vi "detect circles 4.vi"() -> ()   [LabVIEW 2020]
uses:
  <vilib>/vision/NI_Vision_Development_Module.lvlib
panel:
  out "Distances":sgl[](array[numeric]) format="%.4f"
  out "min value":dbl
  out "Array 2":dbl[](array[numeric])
  out "Array":cdb[](array[numeric])
  out "Coordinates":i32[](array[numeric])
  out "Last Mouse Position:All Elements":cluster{"X":i32, "Y":i32}
  out "Circles Data (calibrated)":T1(array[cluster])
  in  "Operation":T2(ring)
  out "Circles Data 2":T1(array[cluster])
  out "error out":errorcluster
  out "Image IN 3":T3(plugin-control)
  in  "WindowSize":i32=9
  in  "LThres":sgl=0.2
  in  "HThresh":sgl=0.7
  in  "Sigma":sgl=1.0
  out "Circles Data":T1(array[cluster])
  in  "Detect circles":bool
  out "Y Resolution":i32
  out "X Resolution":i32
  out "Unit":T4
  out "Image Type":T5 items=["Grayscale (U8)", "Grayscale (I16)", "Grayscale (SGL)", "Complex (CSG)", "RGB (U32)", "HSL (U32)", "RGB (U64)", "Grayscale (U16)"]
  out "Image IN 2":T3(plugin-control)
  out "Image IN":T3(plugin-control)
  in  "Vertical Pointer Slide":cluster{"Numeric":dbl, "Numeric":dbl}(slide)={"Numeric"=0.0, "Numeric"=2.7353463587921847} scale=0.0..255.0
  in  "stop":bool
  in  "Image Type (Conversion 1)":T5 items=["Grayscale (U8)", "Grayscale (I16)", "Grayscale (SGL)", "Complex (CSG)", "RGB (U32)", "HSL (U32)", "RGB (U64)", "Grayscale (U16)"]
  in  "Bit Depth (Original Image)":u32=15
  in  "error in":errorcluster
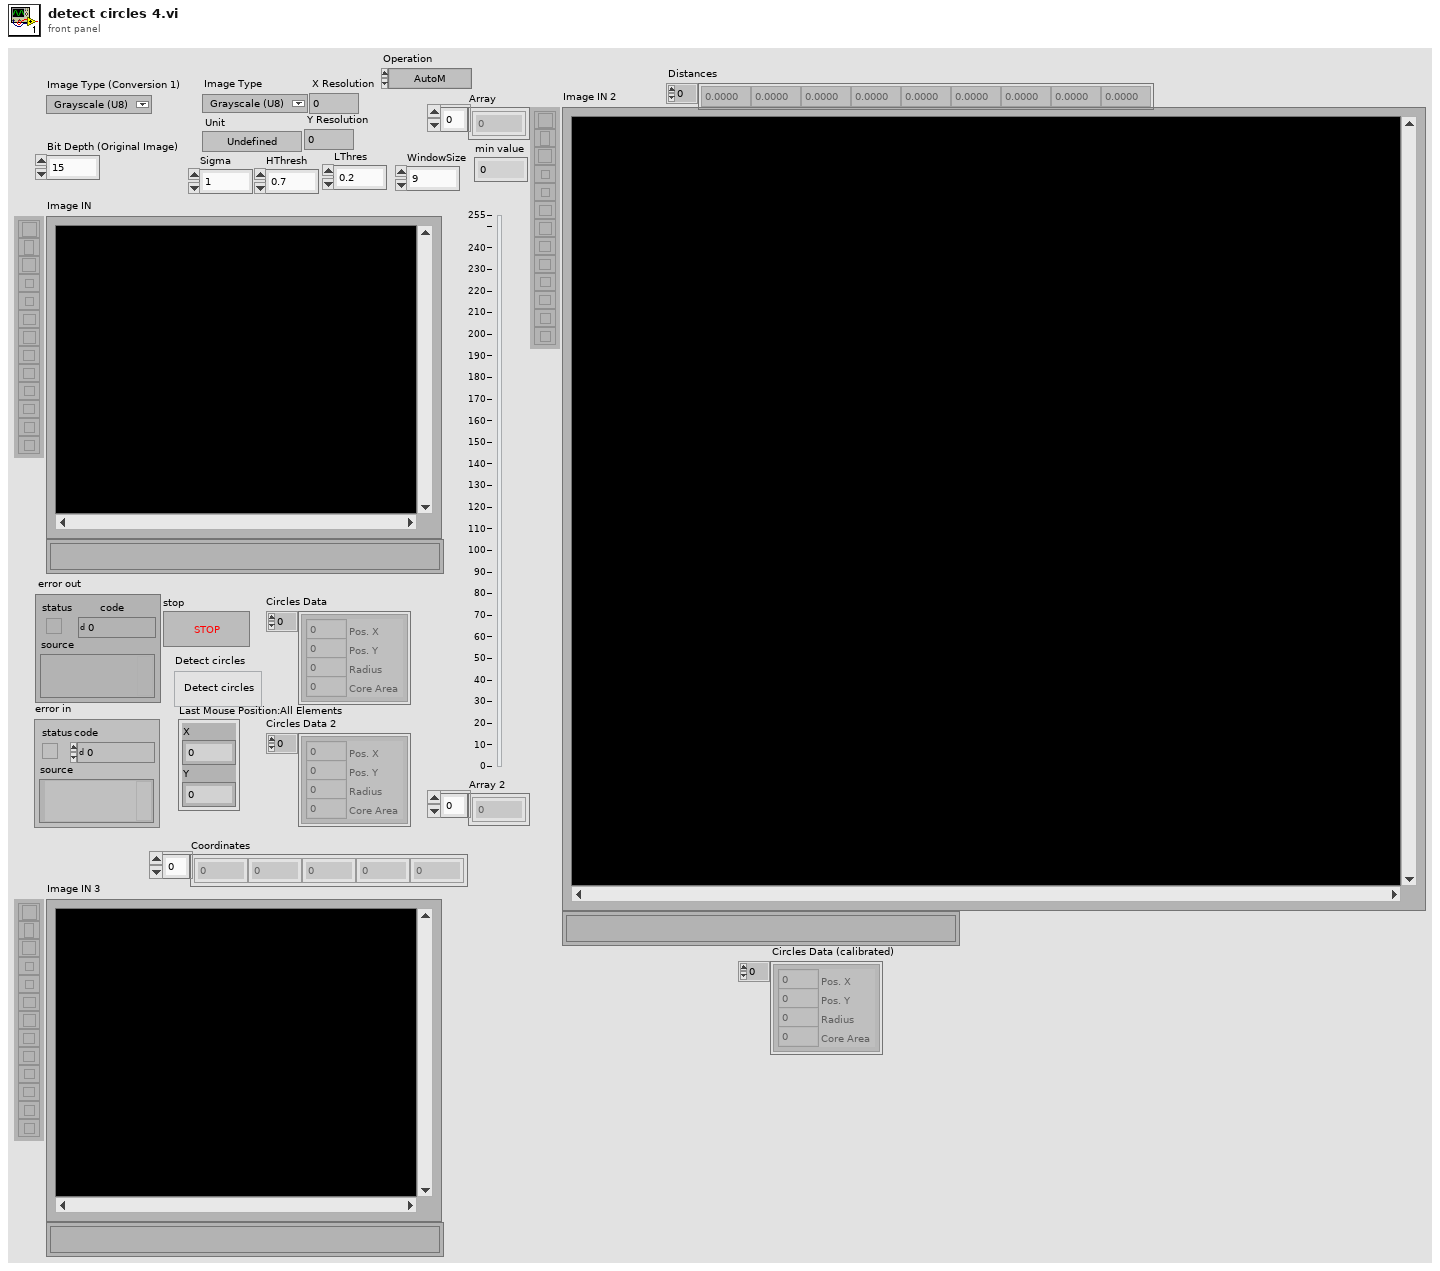
[diagram p1: front panel]
types:
  T1 = cluster{"Pos. X":i32, "Pos. Y":i32, "Radius":i32, "Core Area":i32}[]
  T2 = enum32{"AutoM", "Close", "Dilate", "Erode", "Gradient", "Gradient out", "Gradient in", "Hit miss", "Open", "PClose", "POpen", "Thick", "Thin"}
  T3 = typedef "IMAQ Image.ctl" = refnum<image>
  T4 = typedef "Image Unit" = enum32{"Undefined", "Angström", "Micrometer", "Millimeter", "Centimeter", "Meter", "Kilometer", "Microinch", "Inch", "Feet", "Nautical miles", "Standard miles", "Steps"}
  T5 = typedef "Image Type" = u32
  T6 = cluster{"Conversion Method":u32, "Minimum Value":i32, "Maximum Value":i32, "Number Of Shifts":i32}
  T7 = typedef "IMAQ Circle" = cluster{"Center X":i32, "Center Y":i32, "Inner Radius":i32, "Outer Radius":i32, "Start Angle":dbl, "End Angle":dbl}
  T8 = typedef "IMAQ Point" = cluster{"X":sgl, "Y":sgl}
  T9 = typedef "ROI Descriptor" = cluster{"Global Rectangle":i32[], "Contours":cluster{"ID":enum32{"External", "Internal"}, "Type":u32, "Coordinates":i32[]}[]}
  T10 = cluster{"Pos. X":i32, "Pos. Y":i32, "Radius":i32, "Core Area":i32}
  T11 = cluster{"Sigma":sgl, "HThresh":sgl, "LThres":sgl, "WindowSize":i32}
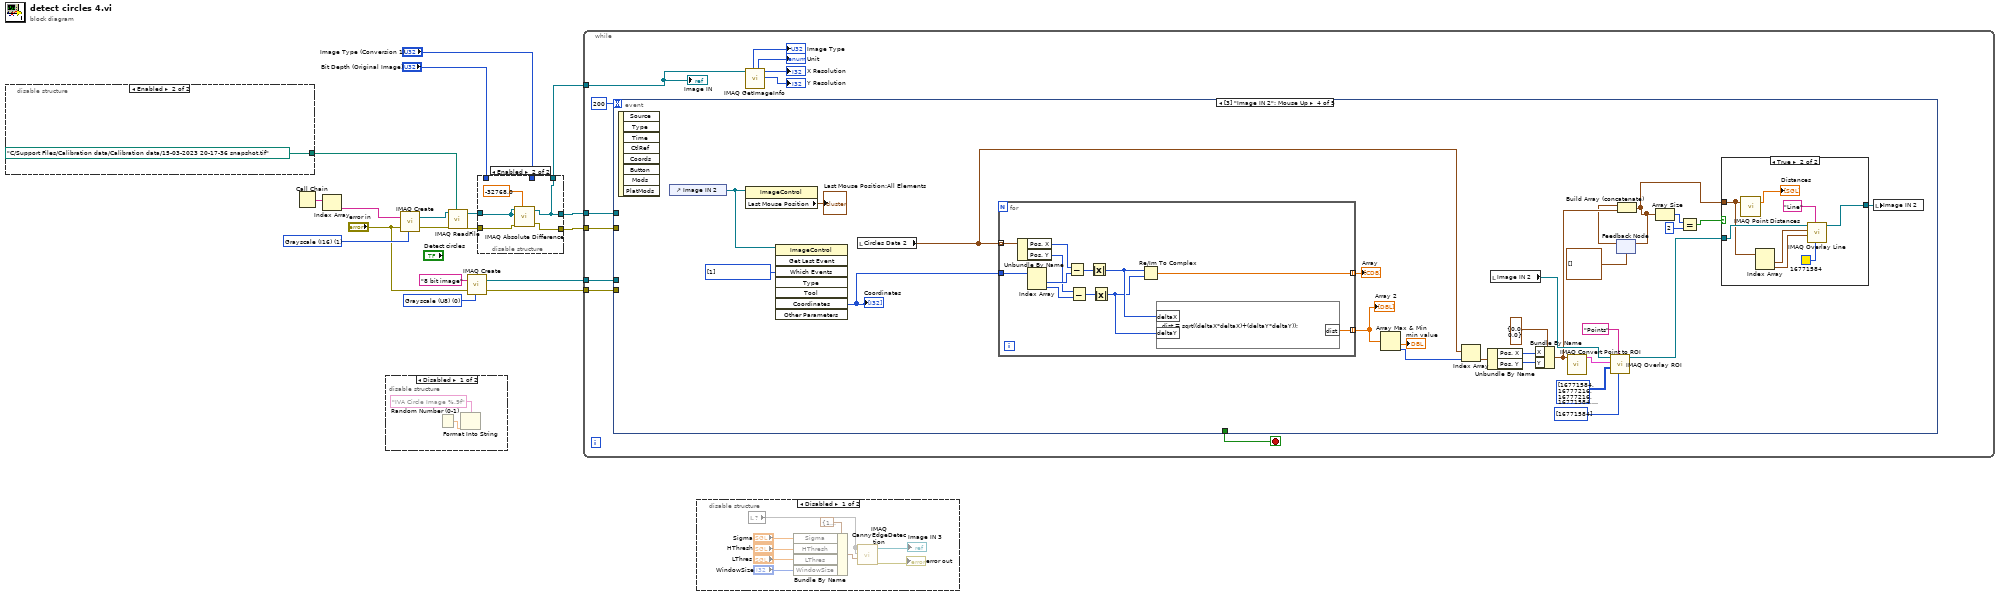
[diagram p0: block diagram]
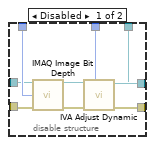
[diagram p3: hidden frame]
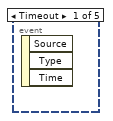
[diagram p4: hidden frame]
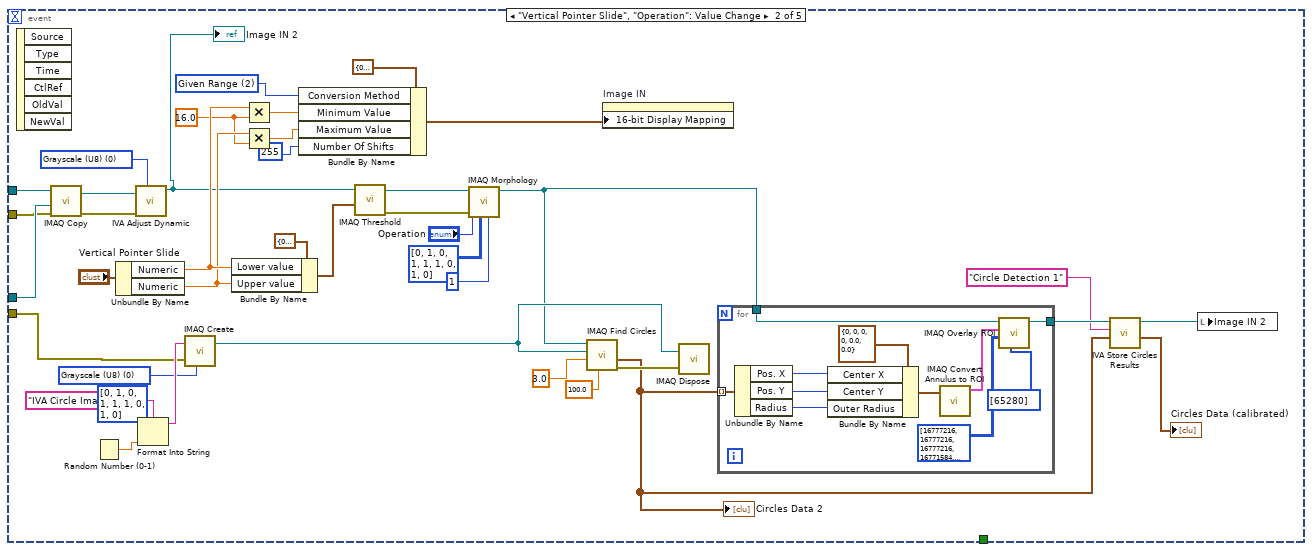
[diagram p5: hidden frame]
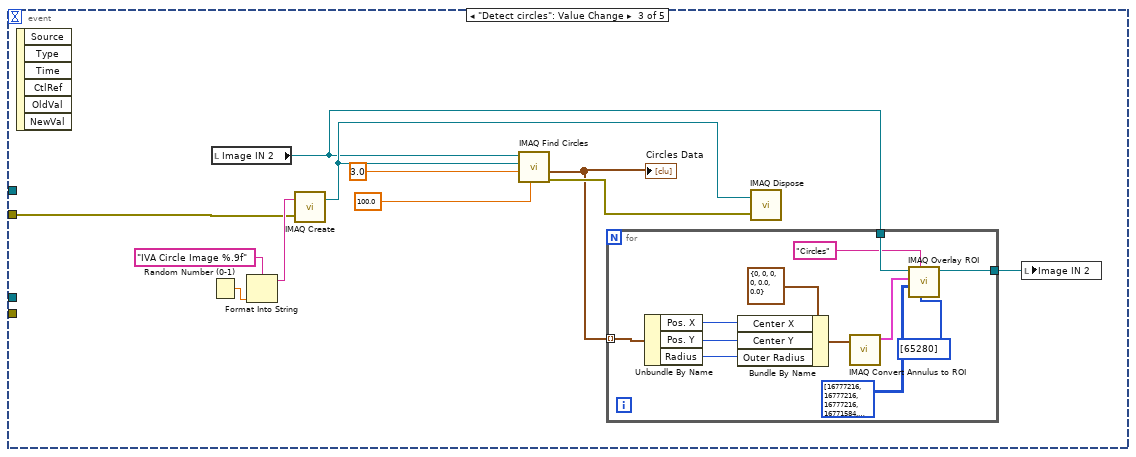
[diagram p6: hidden frame]
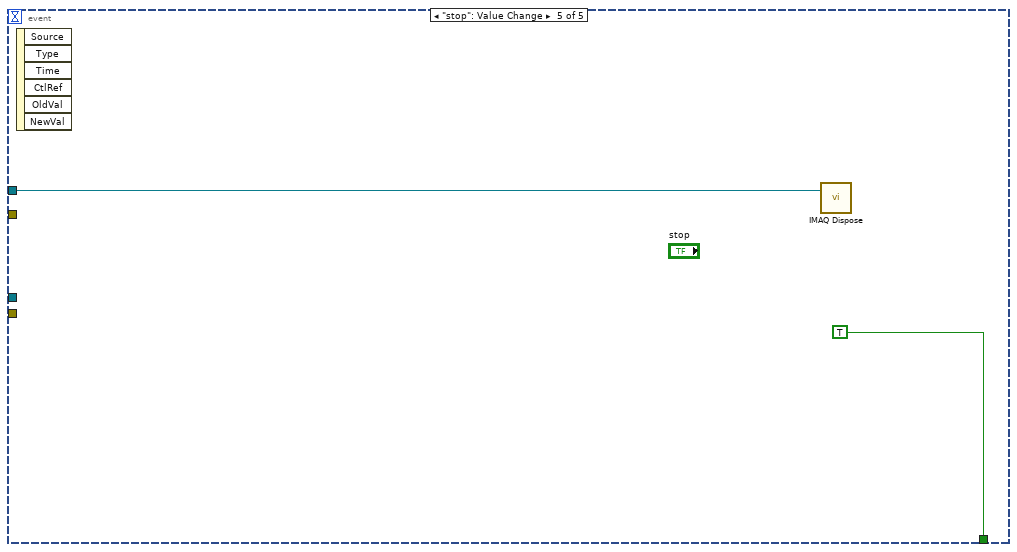
[diagram p8: hidden frame]
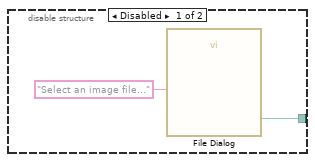
[diagram p10: hidden frame]
diagram:
  w6 = T5 0 items=["Grayscale (U8)", "Grayscale (I16)", "Grayscale (SGL)", "Complex (CSG)", "RGB (U32)", "HSL (U32)", "RGB (U64)", "Grayscale (U16)"] ("Image Type")
  w13 = T5 1 items=["Grayscale (U8)", "Grayscale (I16)", "Grayscale (SGL)", "Complex (CSG)", "RGB (U32)", "HSL (U32)", "RGB (U64)", "Grayscale (U16)"] ("Image Type")
  n1 = disable-structure shown="Enabled" {
    disable-tunnel: [w19 path "C:/Support Files/Calibration data/Calibration data/15-03-2023 20-17-36 snapshot.tif" ("File Path")] -> w14
    frame Disabled {
      n2 = call "File Dialog"("prompt"="Select an image file...") -> ("selected path"=w19:path)  [unwired: 6 in, 8 out]
    }
    frame Enabled {
    }
  }
  n3 = Call Chain() -> (call chain=w16:string[])
  n4 = Index Array(array=w16) -> (element=w15:string)  [unwired: 1 in]
  n5 = disable-structure shown="Disabled" {
    frame Disabled {
      n6 = Random Number (0-1)() -> (number: 0 to 1=w22:dbl)
      n7 = Format Into String(format string="IVA Circle Image %.9f" ("Image Name"), w22) -> ()  [unwired: 2 in, 2 out]
    }
    frame Enabled {
    }
  }
  n8 = call "IMAQ Create"("Image Name"=w15, "Image Type"=w13, "error in (no error)"="error in") -> ("New Image"=w18:T3, "error out"=w17:errorcluster)  [unwired: 1 in, 1 out]
  n9 = call "IMAQ ReadFile"("File Path"=w14, "error in (no error)"=w17, "Image"=w18) -> ("error out"=w10:errorcluster, "Image Out"=w11:T3)  [unwired: 2 in, 5 out]
  n10 = call "IMAQ Create"("Image Name"="8 bit image", "Image Type"=w6, "error in (no error)"="error in") -> ("New Image"=w3:T3, "error out"=w8:errorcluster)  [unwired: 1 in, 1 out]
  n11 = disable-structure shown="Enabled" {
    disable-tunnel: "Bit Depth (Original Image)" -> [w31 _]
    disable-tunnel: w11 -> [w30 w34]
    disable-tunnel: w10 -> [w29 w35]
    disable-tunnel: "Image Type (Conversion 1)" -> [w28 _]
    disable-tunnel: [w26 w32] -> w5
    disable-tunnel: [w25 w33] -> w4
    disable-tunnel: [w24 w32] -> w2
    frame Disabled {
      n12 = call "IMAQ Image Bit Depth"("Image"=w30, "Bit Depth (0)"=w31, "error in (no error)"=w29) -> ("Image Out"=w24:T3, "error out"=w27:errorcluster)  [unwired: 10 in, 1 out]
      n13 = call <vilib>:"IVA Adjust Dynamic.vi"("Image Type"=w28, "error in (no error)"=w27, "Image Src"=w24) -> ("error out"=w25:errorcluster, "Image Out"=w26:T3)  [unwired: 7 out]
    }
    frame Enabled {
      n14 = call "IMAQ Absolute Difference"("Image Src A"=w34, "Constant"=-32768.0, "Image Dst"=w34, "error in (no error)"=w35) -> ("Image Dst Out"=w32:T3, "error out"=w33:errorcluster)  [unwired: 3 in]
    }
  }
  n15 = while {
    tunnel: w4 -> [w44]
    tunnel: w8 -> [w47]
    tunnel: w5 -> [w42]
    tunnel: w3 -> [w43]
    tunnel: w2 -> [w41]
    stop <- w45 stop-if-true
    n16 = event shown="[3] \"Image IN 2\": Mouse Up" {
      selector: _ -> [_ _ _ _ _]
      dyn-events: _ -> [_ _ _ _ _]
      timeout: 200 -> [_ _ _ _ _]
      tunnel: w44 -> [_ w78 w105 _ _]
      tunnel: w42 -> [_ w68 _ _ w169]
      tunnel: w47 -> [_ w64 _ _ _]
      tunnel: [_ _ _ _ TRUE ("stop")] -> w45
      tunnel: w43 -> [_ w79 _ _ _]
      event Timeout {
        n17 = event-data() -> ()  [unwired: 1 in, 3 out]
      }
      event "Vertical Pointer Slide", "Operation": Value Change {
        (unwired) i32[][] [[0, 1, 0], [1, 1, 1], [0, 1, 0]] ("Structuring Element (Basic Morphology 1) 2")
        w63 = T5 0 items=["Grayscale (U8)", "Grayscale (I16)", "Grayscale (SGL)", "Complex (CSG)", "RGB (U32)", "HSL (U32)", "RGB (U64)", "Grayscale (U16)"] ("Image Type")
        w70 = T5 0 items=["Grayscale (U8)", "Grayscale (I16)", "Grayscale (SGL)", "Complex (CSG)", "RGB (U32)", "HSL (U32)", "RGB (U64)", "Grayscale (U16)"] ("Image Type")
        w73 = 16.0 ("y")
        w81 = u32 2 items=["Full Dynamic", "Downshift", "Given Range", "90% Dynamic", "Given Percent Range"] ("Conversion Method (Given Range)")
        n18 = event-data() -> ()  [unwired: 1 in, 6 out]
        n19 = call "IMAQ Copy"("error in (no error)"=w78, "Image Dst"=w79, "Image Src"=w68) -> ("error out"=w72:errorcluster, "Image Dst Out"=w71:T3)  [unwired: 3 in]
        n20 = Random Number (0-1)() -> (number: 0 to 1=w65:dbl)
        n21 = Unbundle By Name("Vertical Pointer Slide") -> ("Numeric"=w77:dbl, "Numeric"=w74:dbl)
        n22 = call <vilib>:"IVA Adjust Dynamic.vi"("Image Type"=w70, "error in (no error)"=w72, "Image Src"=w71) -> ("Image Out"=w69:T3)  [unwired: 8 out]
        "Image IN 2" <- w69
        n23 = Format Into String(format string="IVA Circle Image %.9f" ("Image Name"), w65) -> (resulting string=w67:string)  [unwired: 2 in, 1 out]
        n24 = call "IMAQ Create"("Image Name"=w67, "Image Type"=w63, "error in (no error)"=w64) -> ("New Image"=w59:T3)  [unwired: 1 in, 2 out]
        n25 = Bundle By Name(cluster=cluster{"Lower value":sgl, "Upper value":sgl} {"Lower value"=0.0, "Upper value"=0.0} ("Range (Threshold 1)"), "Lower value"=w77, "Upper value"=w74) -> (w86:cluster{"Lower value":sgl, "Upper value":sgl})
        n26 = Multiply(x=w77, y=w73) -> (x*y=w76:dbl)
        n27 = Multiply(x=w74, y=w73) -> (x*y=w75:dbl)
        n28 = Bundle By Name(cluster=T6 {"Conversion Method"=0, "Minimum Value"=0, "Maximum Value"=0, "Number Of Shifts"=0} ("16-bit Display Mapping:All Elements"), "Conversion Method"=w81, "Minimum Value"=w76, "Maximum Value"=w75, "Number Of Shifts"=255) -> (w82:T6)
        n29 = call "IMAQ Threshold"("Range"=w86, "Image Src"=w69) -> ("error out"=w58:errorcluster, "Image Dst Out"=w57:T3)  [unwired: 4 in, 4 out]
        n30 = call "IMAQ Morphology"("Number of iterations (1)"=1, "Structuring Element"=i32[][] [[0, 1, 0], [1, 1, 1], [0, 1, 0]] ("Structuring Element (Basic Morphology 1) 2"), "error in (no error)"=w58, "Operation"="Operation", "Image Src"=w57) -> ("Image Dst Out"=w56:T3)  [unwired: 2 in, 4 out]
        n31 = call "IMAQ Find Circles"("Max Radius"=sgl 100.0, "Min Radius"=sgl 3.0, "Image Dst"=w59, "Image Src"=w56) -> ("error out"=w60:errorcluster, "Circles Data"=w50:T1)  [unwired: 1 in, 5 out]
        "Circles Data 2" <- w50
        n32 = property on="Image IN" class="ImageControl"("16-bit Display Mapping"=w82) -> ()  [unwired: 2 in, 2 out]
        n33 = call "IMAQ Dispose"("Image"=w59, "error in (no error)"=w60) -> ()  [unwired: 1 in, 4 out]
        n34 = for {
          tunnel: w50 -> [w96] mode=indexing
          tunnel: w56 -> [w91]
          tunnel: [w87] -> w52
          n35 = Unbundle By Name(w96) -> ("Pos. X"=w95:i32, "Pos. Y"=w94:i32, "Radius"=w93:i32)
          n36 = Bundle By Name(cluster=T7 {"Center X"=0, "Center Y"=0, "Inner Radius"=0, "Outer Radius"=0, "Start Angle"=0.0, "End Angle"=0.0} ("Annulus"), "Center X"=w95, "Center Y"=w94, "Outer Radius"=w93) -> (w92:T7)
          n37 = call "IMAQ Convert Annulus to ROI"("Annulus"=w92) -> ("ROI Descriptor"=w90:T9)  [unwired: 8 in, 1 out]
          n38 = call "IMAQ Overlay ROI"("Colors (Green)"=u32[] [65280], "Point Symbol"=u32[][] [[16777216, 16777216, 16777216, 16771584, 16777216, 16777216, 16777216], [16777216, 16777216, 16777216, 16771584, 16777216, 16777216, 16777216], [16777216, 16777216, 16777216, 16771584, 16777216, 16777216, 16777216], [16771584, 16771584, 16771584, 16771584, 16771584, 16771584, 16771584], [16777216, 16777216, 16777216, 16771584, 16777216, 16777216, 16777216], [16777216, 16777216, 16777216, 16771584, 16777216, 16777216, 16777216], [16777216, 16777216, 16777216, 16771584, 16777216, 16777216, 16777216]], "ROI Descriptor"=w90, "Image"=w91) -> ("Image Out"=w87:T3)  [unwired: 6 in, 1 out]
        }
        n39 = call <vilib>:"IVA Store Circles Results.vi"("Circles Data"=w50, "Step Name"="Circle Detection 1", "Image in"=w52) -> ("Circles Data (calibrated)"=→"Circles Data (calibrated)":T1, "Image dup"=w49:T3)  [unwired: 1 in, 6 out]
        n40 = local write "Image IN 2"(w49) -> ()
      }
      event "Detect circles": Value Change {
        n41 = event-data() -> ()  [unwired: 1 in, 6 out]
        n42 = Random Number (0-1)() -> (number: 0 to 1=w106:dbl)
        n43 = local read "Image IN 2"() -> (w99:T3)
        n44 = Format Into String(format string="IVA Circle Image %.9f" ("Image Name"), w106) -> (resulting string=w108:string)  [unwired: 2 in, 1 out]
        n45 = call "IMAQ Create"("Image Name"=w108, "error in (no error)"=w105) -> ("New Image"=w104:T3)  [unwired: 2 in, 2 out]
        n46 = call "IMAQ Find Circles"("Max Radius"=sgl 100.0, "Min Radius"=sgl 3.0, "Image Dst"=w104, "Image Src"=w99) -> ("error out"=w103:errorcluster, "Circles Data"=w100:T1)  [unwired: 1 in, 5 out]
        "Circles Data" <- w100
        n47 = for {
          tunnel: w100 -> [w119] mode=indexing
          tunnel: w99 -> [w114]
          tunnel: [w110] -> w98
          n48 = Unbundle By Name(w119) -> ("Pos. X"=w118:i32, "Pos. Y"=w117:i32, "Radius"=w116:i32)
          n49 = Bundle By Name(cluster=T7 {"Center X"=0, "Center Y"=0, "Inner Radius"=0, "Outer Radius"=0, "Start Angle"=0.0, "End Angle"=0.0} ("Annulus"), "Center X"=w118, "Center Y"=w117, "Outer Radius"=w116) -> (w115:T7)
          n50 = call "IMAQ Convert Annulus to ROI"("Annulus"=w115) -> ("ROI Descriptor"=w113:T9)  [unwired: 8 in, 1 out]
          n51 = call "IMAQ Overlay ROI"("Colors (Green)"=u32[] [65280], "Group"="Circles", "Point Symbol"=u32[][] [[16777216, 16777216, 16777216, 16771584, 16777216, 16777216, 16777216], [16777216, 16777216, 16777216, 16771584, 16777216, 16777216, 16777216], [16777216, 16777216, 16777216, 16771584, 16777216, 16777216, 16777216], [16771584, 16771584, 16771584, 16771584, 16771584, 16771584, 16771584], [16777216, 16777216, 16777216, 16771584, 16777216, 16777216, 16777216], [16777216, 16777216, 16777216, 16771584, 16777216, 16777216, 16777216], [16777216, 16777216, 16777216, 16771584, 16777216, 16777216, 16777216]], "ROI Descriptor"=w113, "Image"=w114) -> ("Image Out"=w110:T3)  [unwired: 5 in, 1 out]
        }
        n52 = call "IMAQ Dispose"("Image"=w104, "error in (no error)"=w103) -> ()  [unwired: 1 in, 4 out]
        n53 = local write "Image IN 2"(w98) -> ()
      }
      event "Image IN 2": Mouse Up {
        w145 = i32[] [1] items=["No Event"=0, "Click Event"=1, "Draw Event"=2, "Size Event"=4, "Scroll Event"=5, "Double Click Event"=8] ("Which Events")
        n54 = event-data() -> ()  [unwired: 1 in, 8 out]
        n55 = control-ref of="Image IN 2"() -> (w146:refnum<vi>)
        n56 = property class="ImageControl"(reference=w146) -> ("Last Mouse Position"=→"Last Mouse Position:All Elements":cluster{"X":i32, "Y":i32})  [unwired: 1 in, 2 out]
        n57 = invoke class="ImageControl" method="Get Last Event"(reference=w146, "Which Events"=w145) -> ("Coordinates"=w144:i32[])  [unwired: 6 in, 7 out]
        "Coordinates" <- w144
        n58 = local read "Circles Data 2"() -> (w136:T1)
        n59 = for {
          tunnel: w136 -> [w168] mode=indexing
          tunnel: w144 -> [w167]
          tunnel: [w162] -> w142 mode=indexing
          tunnel: [w161] -> w143 mode=indexing
          n60 = Unbundle By Name(w168) -> ("Pos. X"=w160:i32, "Pos. Y"=w158:i32)
          n61 = Index Array(array=w167) -> (element #1=w159:i32, element #2=w157:i32)  [unwired: 2 in]
          n62 = Subtract(x=w160, y=w159) -> (x-y=w166:i32)
          n63 = Subtract(x=w158, y=w157) -> (x-y=w165:i32)
          n64 = Absolute Value(x=w166) -> (abs(x)=w164:i32)
          n65 = Absolute Value(x=w165) -> (abs(x)=w163:i32)
          n66 = Re/Im To Complex(1:w163, 2:w164) -> (0:w161:cdb)
          n67 = formula code="dist = sqrt((deltaX*deltaX)+(deltaY*deltaY));"("deltaX"=w164, "deltaY"=w163) -> ("dist"=w162:dbl)
        }
        "Array" <- w143
        "Array 2" <- w142
        n68 = Array Max & Min(array=w142) -> (min value=→"min value":dbl, min index (indices)=w140:i32)  [unwired: 2 out]
        n69 = Index Array(array=w136, index=w140) -> (element=w139:T10)
        n70 = Unbundle By Name(w139) -> ("Pos. X"=w138:i32, "Pos. Y"=w137:i32)
        n71 = local read "Image IN 2"() -> (w133:T3)
        n72 = Bundle By Name(cluster=T8 {"X"=0.0, "Y"=0.0} ("Point"), "X"=w138, "Y"=w137) -> (w129:T8)
        n73 = call "IMAQ Convert Point to ROI"("Point"=w129) -> ("ROI Descriptor"=w134:T9)  [unwired: 8 in, 1 out]
        n74 = call "IMAQ Overlay ROI"("Colors (Green)"=u32[] [16771584], "Group"="Points", "Point Symbol"=u32[][] [[16771584, 16777216, 16777216, 16771584, 16777216, 16777216, 16771584], [16777216, 16771584, 16777216, 16771584, 16777216, 16771584, 16777216], [16777216, 16777216, 16771584, 16771584, 16771584, 16777216, 16777216], [16771584, 16771584, 16771584, 16771584, 16771584, 16771584, 16771584], [16777216, 16777216, 16771584, 16771584, 16771584, 16777216, 16777216], [16777216, 16771584, 16777216, 16771584, 16777216, 16771584, 16777216], [16771584, 16777216, 16777216, 16771584, 16777216, 16777216, 16771584]], "ROI Descriptor"=w134, "Image"=w133) -> ("Image Out"=w122:T3)  [unwired: 5 in, 1 out]
        n75 = feedback #1(T8[] []) -> (w126:T8[])
        n76 = Build Array (concatenate)(w126, w129) -> (w124:T8[])
        n77 = feedback-in #1(w124) -> ()
        n78 = Array Size(array=w124) -> (size(s)=w128:i32)
        n79 = Equal?(x=w128, y=2) -> (x = y?=w123:bool)
        n80 = case shown="True" w123 {
          tunnel: w124 -> [_ w152]
          tunnel: w122 -> [w148 w155]
          tunnel: [w148 w154] -> w121
          frame False {
          }
          frame True {
            n81 = call "IMAQ Point Distances"("Points"=w152) -> ("Distances"=→"Distances":sgl[])  [unwired: 4 in, 1 out]
            n82 = Index Array(array=w152) -> (element #1=w151:T8, element #2=w150:T8)  [unwired: 2 in]
            n83 = call "IMAQ Overlay Line"("Color"=u32 16771584, "Group"="Line", "End Point"=w150, "Start Point"=w151, "Image"=w155) -> ("Image Out"=w154:T3)  [unwired: 5 in, 1 out]
          }
        }
        n84 = local write "Image IN 2"(w121) -> ()
      }
      event "stop": Value Change {
        n85 = event-data() -> ()  [unwired: 1 in, 6 out]
        n86 = call "IMAQ Dispose"("Image"=w169) -> ()  [unwired: 5 in, 1 out]
      }
    }
    n87 = call "IMAQ GetImageInfo"("Image"=w41) -> ("Y Resolution"=→"Y Resolution":i32, "X Resolution"=→"X Resolution":i32, "Unit"=→"Unit":T4, "Image Type"=→"Image Type":T5)  [unwired: 3 in, 4 out]
    "Image IN" <- w41
  }
  n88 = disable-structure shown="Disabled" {
    frame Disabled {
      n89 = local read item#-1() -> (w178)
      n90 = Bundle By Name(cluster=T11 {"Sigma"=1.0, "HThresh"=0.7, "LThres"=0.2, "WindowSize"=9} ("Filter Parameters"), "Sigma"="Sigma", "HThresh"="HThresh", "LThres"="LThres", "WindowSize"="WindowSize") -> (w172:T11)
      n91 = call "IMAQ CannyEdgeDetection"("Image Src"=w178, "Image Dst"=w178, "Filter Parameters"=w172) -> ("Image Dst Out"=→"Image IN 3":T3, "error out"=→"error out":errorcluster)  [unwired: 5 in]
    }
    frame Enabled {
    }
  }
